vi "Get Biometry Data.vi"(8 "error in (no error)":errorcluster caption="错误输入（无错误）", 9 "Display Parameter":T1(ring), 10 "condition":string, 11 "connection reference":T2) -> (0 "error out":errorcluster caption="错误输出", 2 "Data Output":string[][](array[string]))   [LabVIEW 2015, in "Utility VIs.lvlib"]
doc: "该模板用于创建子VI。"
uses:
  Utility VIs.lvlib
  <vilib>/addons/database/Connection.llb/Conn ObjectReference.ctl
  Database Processing/Database Processing.lvlib
  <vilib>/addons/database/NI_Database_API.lvlib
panel:
  # "Busy"
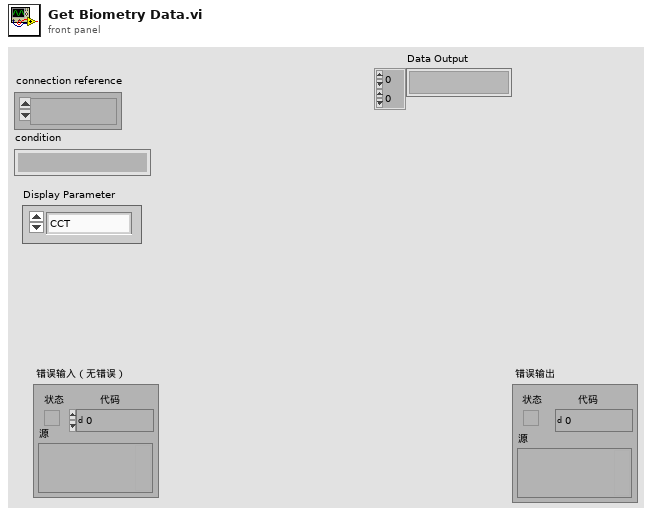
[diagram p1: front panel]
types:
  T1 = enum16{"CCT", "ACD", "LT", "RT", "AL", "PD", "WTW", "K_flat", "K_steep"}
  T2 = typedef "NI_Database_API.lvlib/Conn ObjectReference.ctl" = refnum<k1>
  T3 = typedef "Database Processing.lvlib/Biometry Attribute.ctl" = cluster{"Measure_ID":i64, "Measure_No":i64, "Ordinal":i64, "L_Or_R":string}
  T4 = typedef "Database Processing.lvlib/Biometry Parameter.ctl" = cluster{"Measure_ID":i64, "Central_Corneal_Thickness":sgl, "Anterior_Chamber_Depth":sgl, "Len_Thickness":sgl, "Retinal_Thickness":sgl, "Axis_Length":sgl, "Pupil_Diameter":sgl, "PCX":sgl, "PCY":sgl, "White_To_White":sgl, "ICX":sgl, "ICY":sgl, "Keratometric_flat":sgl, "Keratometric_steep":sgl, "Keratometric_Axis(flat)":sgl, "Keratometric_Axis(steep)":sgl, "Keratometric_AST":sgl}
  T5 = typedef "Database Processing.lvlib/Biometry State.ctl" = cluster{"Measure_ID":i64, "Central_Corneal_Thickness_State":string, "Anterior_Chamber_Depth_State":string, "Len_Thickness_State":string, "Retinal_Thickness_State":string, "Axis_Length_State":string, "Pupil_Diameter_State":string, "White_To_White_State":string, "Keratometric_flat_State":string, "Keratometric_steep_State":string}
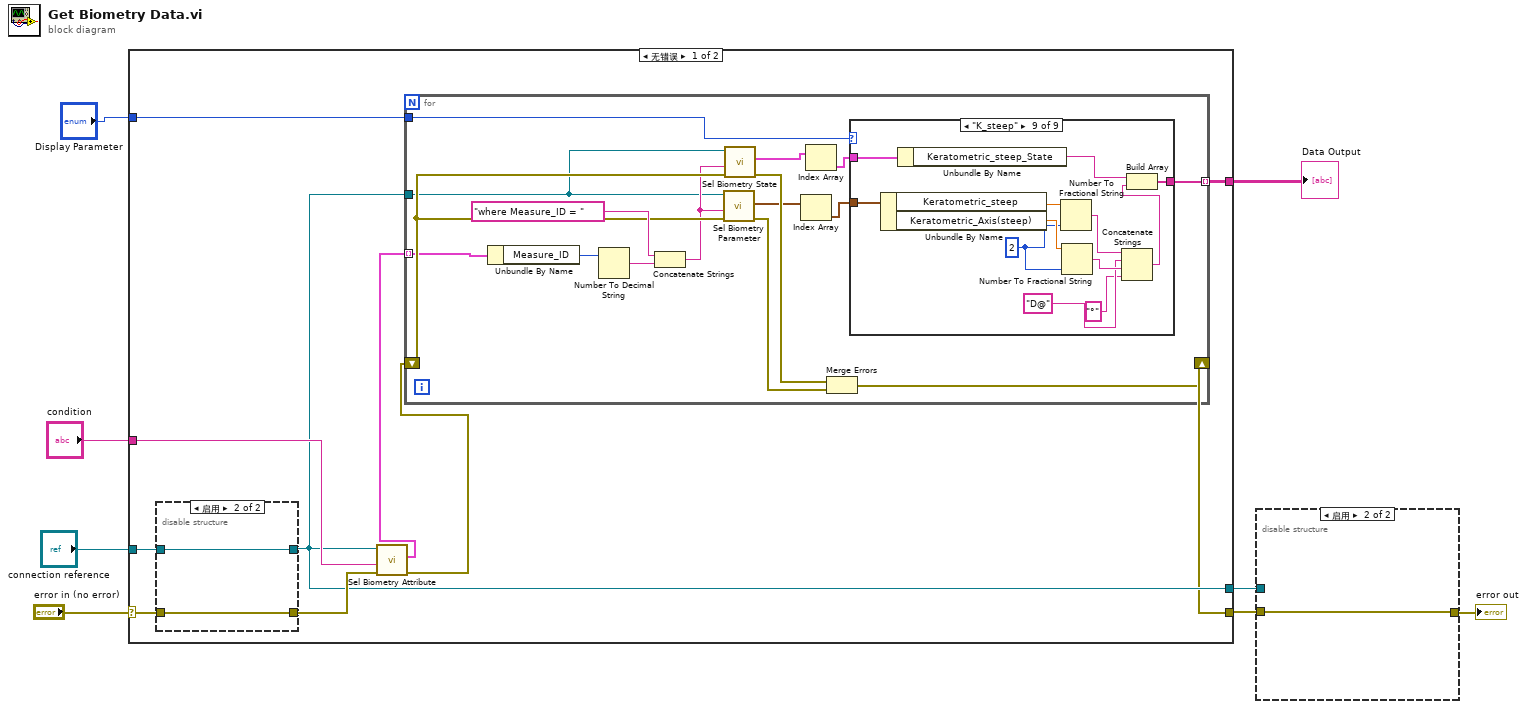
[diagram p0: block diagram]
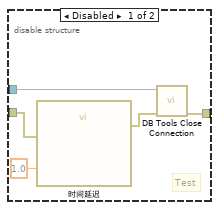
[diagram p2: hidden frame]
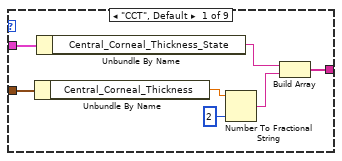
[diagram p3: hidden frame]
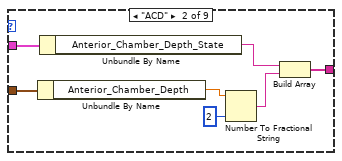
[diagram p4: hidden frame]
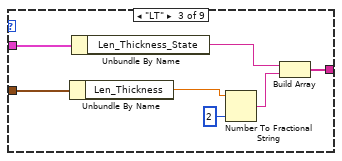
[diagram p5: hidden frame]
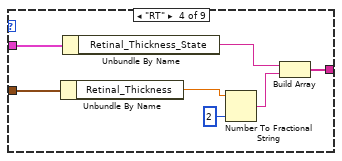
[diagram p6: hidden frame]
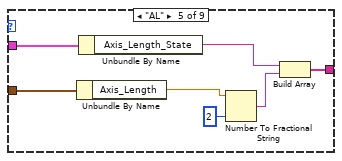
[diagram p7: hidden frame]
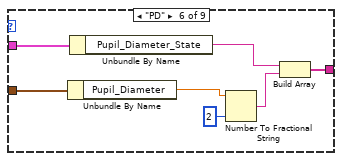
[diagram p8: hidden frame]
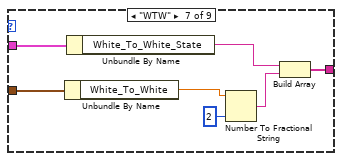
[diagram p9: hidden frame]
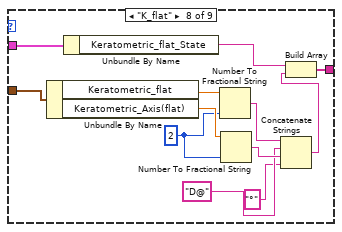
[diagram p10: hidden frame]
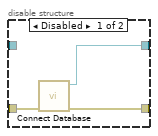
[diagram p11: hidden frame]
diagram:
  n1 = case shown="无错误" "error in (no error)" {
    selector: "error in (no error)" -> [w18 w114]
    tunnel: [w11 w114] -> w5
    tunnel: "connection reference" -> [w17 w113]
    tunnel: "condition" -> [w15 _]
    tunnel: [w13 w113] -> w3
    tunnel: [w12 _] -> w2
    tunnel: "Display Parameter" -> [w10 _]
    frame No Error {
      n2 = disable-structure shown="启用" {
        disable-tunnel: w18 -> [w110 w111]
        disable-tunnel: w17 -> [_ w112]
        disable-tunnel: [w109 w112] -> w13
        disable-tunnel: [w108 w111] -> w16
        frame Disabled {
          n3 = call "Connect Database.vi"("error in (no error)"=w110) -> ("error out"=w108:errorcluster, "connection reference"=w109:T2)  [unwired: 9 in]
        }
        frame Enabled {
        }
      }
      n4 = call "Sel Biometry Attribute.vi"("error in (no error)"=w16, "condition"=w15, "connection reference"=w13) -> ("error out"=w14:errorcluster, "Biometry Attribute"=w9:T3[])  [unwired: 7 in]
      n5 = for {
        tunnel: w13 -> [w29]
        tunnel: [w26] -> w12 mode=indexing
        tunnel: w10 -> [w24]
        shift-right: [w25] -> w11
        shift-left: w14 -> [w31]
        tunnel: w9 -> [w23] mode=indexing
        n6 = Unbundle By Name(w23) -> ("Measure_ID"=w33:i64)
        n7 = Number To Decimal String(number=w33) -> (decimal integer string=w34:string)  [unwired: 1 in]
        n8 = Concatenate Strings("where Measure_ID = " ("字符串"), w34) -> (w30:string)
        n9 = call "Sel Biometry Parameter.vi"("error in (no error)"=w31, "condition"=w30, "connection reference"=w29) -> ("error out"=w27:errorcluster, "Biometry Parameter"=w20:T4[])  [unwired: 7 in]
        n10 = call "Sel Biometry State.vi"("error in (no error)"=w31, "condition"=w30, "connection reference"=w29) -> ("error out"=w28:errorcluster, "Biometry State"=w21:T5[])  [unwired: 7 in]
        n11 = Index Array(array=w20) -> (element=w19:T4)  [unwired: 1 in]
        n12 = Index Array(array=w21) -> (element=w22:T5)  [unwired: 1 in]
        n13 = Merge Errors(w28, w27) -> (w25:errorcluster)
        n14 = case shown="\"K_steep\"" w24 {
          tunnel: w19 -> [w41 w48 w55 w62 w69 w76 w83 w95 w107]
          tunnel: w22 -> [w40 w47 w54 w61 w68 w75 w82 w94 w106]
          tunnel: [w35 w42 w49 w56 w63 w70 w77 w91 w103] -> w26
          frame "CCT", Default {
            n15 = Unbundle By Name(w41) -> ("Central_Corneal_Thickness"=w38:sgl)
            n16 = Unbundle By Name(w40) -> ("Central_Corneal_Thickness_State"=w39:string)
            n17 = Number To Fractional String(number=w38, precision (6)=i16 2 ("精度(6)")) -> (F-format string=w37:string)  [unwired: 2 in]
            n18 = Build Array(w39, w37) -> (w35:string[])
          }
          frame "ACD" {
            n19 = Unbundle By Name(w48) -> ("Anterior_Chamber_Depth"=w45:sgl)
            n20 = Unbundle By Name(w47) -> ("Anterior_Chamber_Depth_State"=w46:string)
            n21 = Number To Fractional String(number=w45, precision (6)=i16 2 ("精度(6)")) -> (F-format string=w44:string)  [unwired: 2 in]
            n22 = Build Array(w46, w44) -> (w42:string[])
          }
          frame "LT" {
            n23 = Unbundle By Name(w55) -> ("Len_Thickness"=w52:sgl)
            n24 = Unbundle By Name(w54) -> ("Len_Thickness_State"=w53:string)
            n25 = Number To Fractional String(number=w52, precision (6)=i16 2 ("精度(6)")) -> (F-format string=w51:string)  [unwired: 2 in]
            n26 = Build Array(w53, w51) -> (w49:string[])
          }
          frame "RT" {
            n27 = Unbundle By Name(w62) -> ("Retinal_Thickness"=w59:sgl)
            n28 = Unbundle By Name(w61) -> ("Retinal_Thickness_State"=w60:string)
            n29 = Number To Fractional String(number=w59, precision (6)=i16 2 ("精度(6)")) -> (F-format string=w58:string)  [unwired: 2 in]
            n30 = Build Array(w60, w58) -> (w56:string[])
          }
          frame "AL" {
            n31 = Unbundle By Name(w69) -> ("Axis_Length"=w66:sgl)
            n32 = Unbundle By Name(w68) -> ("Axis_Length_State"=w67:string)
            n33 = Number To Fractional String(number=w66, precision (6)=i16 2 ("精度(6)")) -> (F-format string=w65:string)  [unwired: 2 in]
            n34 = Build Array(w67, w65) -> (w63:string[])
          }
          frame "PD" {
            n35 = Unbundle By Name(w76) -> ("Pupil_Diameter"=w73:sgl)
            n36 = Unbundle By Name(w75) -> ("Pupil_Diameter_State"=w74:string)
            n37 = Number To Fractional String(number=w73, precision (6)=i16 2 ("精度(6)")) -> (F-format string=w72:string)  [unwired: 2 in]
            n38 = Build Array(w74, w72) -> (w70:string[])
          }
          frame "WTW" {
            n39 = Unbundle By Name(w83) -> ("White_To_White"=w80:sgl)
            n40 = Unbundle By Name(w82) -> ("White_To_White_State"=w81:string)
            n41 = Number To Fractional String(number=w80, precision (6)=i16 2 ("精度(6)")) -> (F-format string=w79:string)  [unwired: 2 in]
            n42 = Build Array(w81, w79) -> (w77:string[])
          }
          frame "K_flat" {
            w89 = i16 2 ("精度(6)")
            n43 = Unbundle By Name(w95) -> ("Keratometric_flat"=w92:sgl, "Keratometric_Axis(flat)"=w90:sgl)
            n44 = Unbundle By Name(w94) -> ("Keratometric_flat_State"=w93:string)
            n45 = Number To Fractional String(number=w92, precision (6)=w89) -> (F-format string=w88:string)  [unwired: 2 in]
            n46 = Number To Fractional String(number=w90, precision (6)=w89) -> (F-format string=w87:string)  [unwired: 2 in]
            n47 = Concatenate Strings(w88, "D@" ("字符串"), w87, "°" ("字符串")) -> (w84:string)
            n48 = Build Array(w93, w84) -> (w91:string[])
          }
          frame "K_steep" {
            w101 = i16 2 ("精度(6)")
            n49 = Unbundle By Name(w107) -> ("Keratometric_steep"=w104:sgl, "Keratometric_Axis(steep)"=w102:sgl)
            n50 = Unbundle By Name(w106) -> ("Keratometric_steep_State"=w105:string)
            n51 = Number To Fractional String(number=w104, precision (6)=w101) -> (F-format string=w100:string)  [unwired: 2 in]
            n52 = Number To Fractional String(number=w102, precision (6)=w101) -> (F-format string=w99:string)  [unwired: 2 in]
            n53 = Concatenate Strings(w100, "D@" ("字符串"), w99, "°" ("字符串")) -> (w96:string)
            n54 = Build Array(w105, w96) -> (w103:string[])
          }
        }
      }
    }
    frame Error {
    }
  }
  "Data Output" <- w2
  n55 = disable-structure shown="启用" {
    disable-tunnel: w5 -> [w117 w120]
    disable-tunnel: [w119 w120] -> w4
    disable-tunnel: w3 -> [w118 _]
    frame Disabled {
      # "Test"
      n56 = call "时间延迟"("error in (no error)"=w117, "Delay Time (s)"=1.0) -> ("error out"=w116:errorcluster)  [unwired: 9 in]
      n57 = call <vilib>:"DB Tools Close Connection.vi"("error in (no error)"=w116, "connection reference"=w118) -> ("error out"=w119:errorcluster)  [unwired: 5 in]
    }
    frame Enabled {
    }
  }
  "error out" <- w4
